vi "Real Compact Cholesky Factor.vi"(0 "Compact Array":cluster{"Compact Array":dbl[], "array type":i32}={"Compact Array"=[], "array type"=2} {"array type" items=["lower triangular", "upper triangular", "symmetric matrix"]; "Compact Array" format="%.2f"}) -> (1 "Cholesky Compact Array":cluster{"Compact Array":dbl[], "array type":i32}={"Compact Array"=[], "array type"=2} {"array type" items=["lower triangular", "upper triangular", "symmetric matrix"]; "Compact Array" format="%.2f"}, 2 "error":i32)   [LabVIEW 2014, in "NI_AALBase.lvlib"]
doc: "Performs the cross multiplication of two input matrices. If A represents the first input matrix, B the second input, and C the resulting output matrix, the elements of C are determined according to the following equation\n\n C[i,j] = Sum{ A[i,l] B[l,j] } for l = 0, 1, 2, ...k-1\n\n where\n k is the number of columns in A and the number of rows in\n B\n j ranges from 0 to (number of columns in B - 1)\n i ranges from 0 to (number of rows in A - 1)."
uses:
  NI_AALBase.lvlib
  lvanlys.dll
panel:
  # "Real Compact Cholseky Factor"
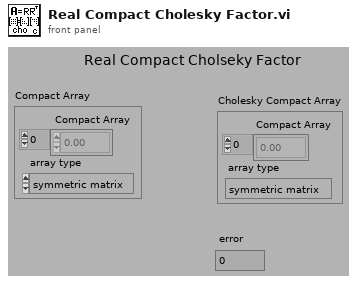
[diagram p1: front panel]
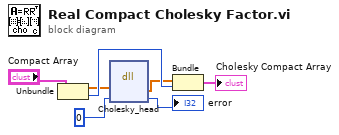
[diagram p0: block diagram]
diagram:
  n1 = Unbundle("Compact Array") -> ("Compact Array"=w5:dbl[], "array type"=w6:i32)
  n2 = dll-call lib="C:/Program Files (x86)/National Instruments/LabVIEW 2014/resource/lvanlys.*" fn="Cholesky_head"("Compact Array"=w5, 0) -> ("Compact Array"=w4:dbl[], →"error":i32)  [unwired: 4 in, 2 out]
  n3 = Bundle("Compact Array"=w4, "array type"=w6) -> (→"Cholesky Compact Array":cluster{"Compact Array":dbl[], "array type":i32})  [unwired: 1 in]
